vi "winForms initColor.vi"(2 "error in (no error)":errorcluster, 3 "Color Box":u32(colorbox)=16448250) -> (0 "error out":errorcluster, 1 "reference out":refnum<k24>)   [LabVIEW 2018]
uses:
  System.Drawing
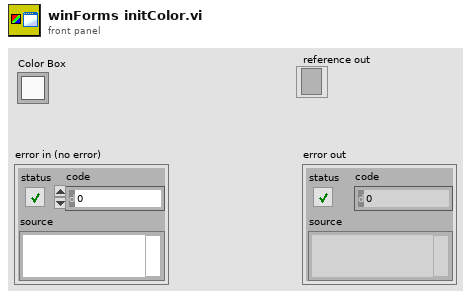
[diagram p1: front panel]
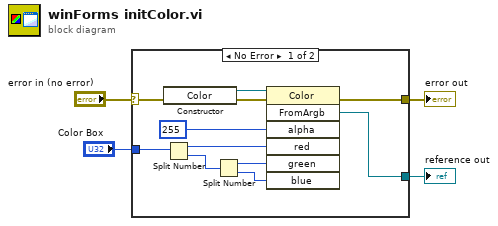
[diagram p0: block diagram]
diagram:
  n1 = case shown="No Error" "error in (no error)" {
    selector: "error in (no error)" -> [w6 w16]
    tunnel: [w8 _] -> w4
    tunnel: "Color Box" -> [w7 _]
    tunnel: [w5 w16] -> w1
    frame No Error {
      n2 = constructor class="Color"(error in=w6) -> (reference out=w14:refnum<k24>, error out=w13:errorcluster)  [unwired: 2 in, 1 out]
      n3 = Split Number(x=w7) -> (hi(x)=w12:u16, lo(x)=w15:u16)
      n4 = Split Number(x=w15) -> (hi(x)=w11:u8, lo(x)=w10:u8)
      n5 = invoke class="Color" method="FromArgb"(reference=w14, error in=w13, "alpha"=255, "red"=w12, "green"=w11, "blue"=w10) -> (error out=w5:errorcluster, "FromArgb"=w8:refnum<k24>)  [unwired: 1 in, 5 out]
    }
    frame Error {
    }
  }
  "reference out" <- w4
  "error out" <- w1
